vi "Attenuator Unflatten Test Parameters.vi"(9 "error in (no error)":errorcluster, 10 "Parameter String":string) -> (1 "error out":errorcluster, 2 "Attenuator Test Parameters":T2={"Stimulus"={"ATT Stimulus"={"Normalize"=TRUE, "Value (dB)"=0.0}, "VNA Stimulus"={"Use Instrument Settings"=FALSE, "Blank Frequencies"=FALSE, "Sweep Type"=enum."Linear", "Sweep"={"Fstart"=500.0, "Fstop"=1500.0, "Units"=enum."MHz", "Points"=201}, "Power (dBm)"=999.0, "IFBW (Hz)"=-1.0, "Sweep Time (s)"=-1.0, "Calibration"={"State"=FALSE, "String"=""}}}, "Measurement"={"Step (dB)"=enum."0.25", "Start (dB)"=0.0, "Stop (dB)"=31.75}, "Limit"={"Maximum Error"=0.3}, "Normalization"={"Normalized?"=FALSE, "Normalization Values (dB)"=[]}} {"Stimulus"."VNA Stimulus"."Sweep Time (s)" format="%.3g"}, 5 "Test Version":string)   [LabVIEW 2011]
uses:
  TypeDefs/Attenuator Test Parameters.ctl
  TypeDefs/Attenuator Stimulus Parameters.ctl
  TypeDefs/Attenuator ATT Stimulus.ctl
  TypeDefs/Attenuator VNA Stimulus.ctl
  S Parameter/TypeDefs/SP Frequency Units.ctl
  TypeDefs/Attenuator VNA Calibration State.ctl
  TypeDefs/Attenuator Measurement Cluster.ctl
  TypeDefs/Attenuator Limit.ctl
  TypeDefs/Attenuator Calibration State.ctl
  Test Return Parameter.ctl
panel:
  in  "Return Parameter":T1
  out "Parameter Variant":variant
  in  "Required Instruments":string[](array[string])=["ATT", "VNA"]
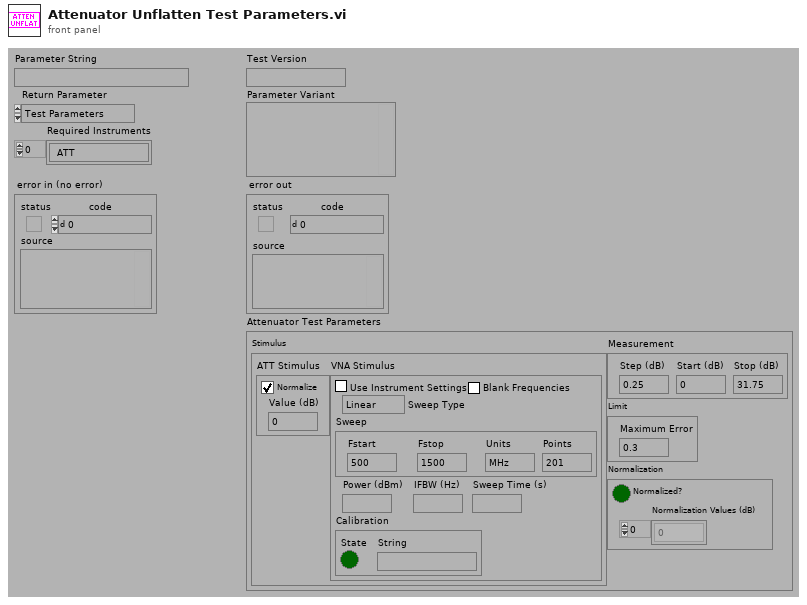
[diagram p1: front panel]
types:
  T1 = typedef "Test Return Parameter.ctl" = enum16{"Test Parameters", "Required Instruments", "Datasheets", "QuickMode"}
  T2 = typedef "Attenuator Test Parameters.ctl" = cluster{"Stimulus":T3, "Measurement":T8, "Limit":T9, "Normalization":T10}
  T3 = typedef "Attenuator Stimulus Parameters.ctl" = cluster{"ATT Stimulus":T4, "VNA Stimulus":T5}
  T4 = typedef "Attenuator ATT Stimulus.ctl" = cluster{"Normalize":bool, "Value (dB)":dbl}
  T5 = typedef "Attenuator VNA Stimulus.ctl" = cluster{"Use Instrument Settings":bool, "Blank Frequencies":bool, "Sweep Type":enum32{"Linear", "Logarithmic", "List", "Power", "CW"}, "Sweep":cluster{"Fstart":dbl, "Fstop":dbl, "Units":T6, "Points":i32}, "Power (dBm)":dbl, "IFBW (Hz)":dbl, "Sweep Time (s)":dbl, "Calibration":T7}
  T6 = typedef "SP Frequency Units.ctl" = enum16{"Hz", "kHz", "MHz", "GHz", "Points"}
  T7 = typedef "Attenuator VNA Calibration State.ctl" = cluster{"State":bool, "String":string}
  T8 = typedef "Attenuator Measurement Cluster.ctl" = cluster{"Step (dB)":enum16{"0.25", "0.50", "1.00"}, "Start (dB)":dbl, "Stop (dB)":dbl}
  T9 = typedef "Attenuator Limit.ctl" = cluster{"Maximum Error":dbl}
  T10 = typedef "Attenuator Calibration State.ctl" = cluster{"Normalized?":bool, "Normalization Values (dB)":dbl[]}
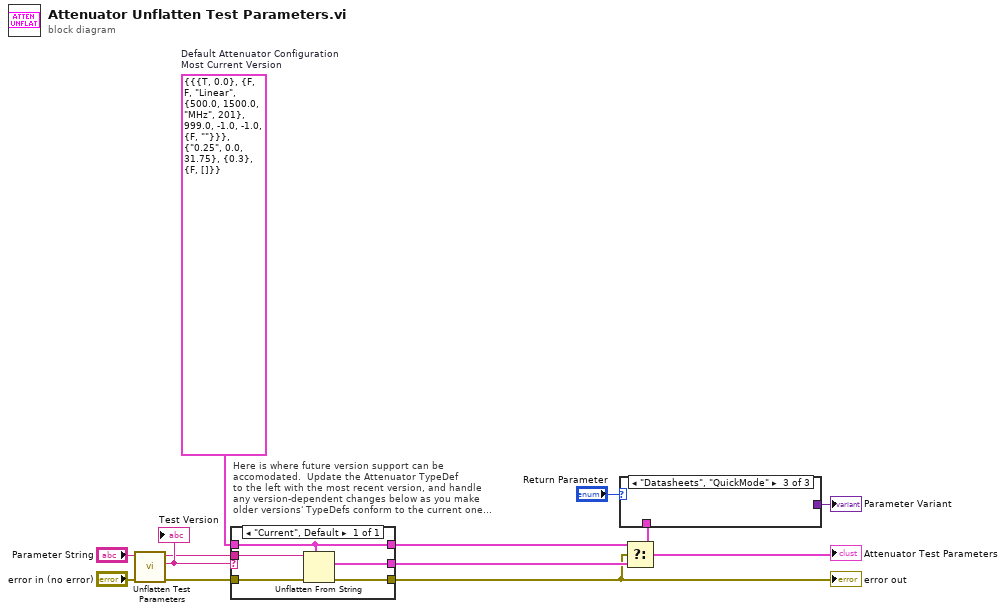
[diagram p0: block diagram]
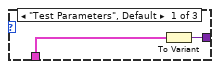
[diagram p2: hidden frame]
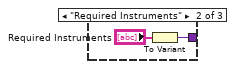
[diagram p3: hidden frame]
diagram:
  w1 = T2 {"Stimulus"={"ATT Stimulus"={"Normalize"=TRUE, "Value (dB)"=0.0}, "VNA Stimulus"={"Use Instrument Settings"=FALSE, "Blank Frequencies"=FALSE, "Sweep Type"=enum."Linear", "Sweep"={"Fstart"=500.0, "Fstop"=1500.0, "Units"=enum."MHz", "Points"=201}, "Power (dBm)"=999.0, "IFBW (Hz)"=-1.0, "Sweep Time (s)"=-1.0, "Calibration"={"State"=FALSE, "String"=""}}}, "Measurement"={"Step (dB)"=enum."0.25", "Start (dB)"=0.0, "Stop (dB)"=31.75}, "Limit"={"Maximum Error"=0.3}, "Normalization"={"Normalized?"=FALSE, "Normalization Values (dB)"=[]}}  # Default Attenuator Configuration Most Current Version
  # "Here is where future version support can be\naccomodated.  Update the Attenuator TypeDef\nto the left with the most recent version, and handle\nany version-dependent changes below as you make\nolder versions' TypeDefs conform to the current one..."
  n1 = call "Unflatten Test Parameters.vi"("error in (no error)"="error in (no error)", "Flattened Test Parameters with Version (\"\")"="Parameter String") -> ("error out"=w3:errorcluster, "Test Version"=w11:string, "Flat Test Parameters"=w10:string)  [unwired: 3 out]
  "Test Version" <- w11
  n2 = case shown="\"Current\", Default" w11 {
    tunnel: [w16] -> w9
    tunnel: w10 -> [w17]
    tunnel: [w14] -> w4
    tunnel: w3 -> [w15]
    tunnel: w1 -> [w13]
    tunnel: [w13] -> w2
    frame "Current", Default {
      n3 = Unflatten From String(type=w13, binary string=w17, error in (no error)=w15) -> (value=w16:T2, error out=w14:errorcluster)  [unwired: 3 out]
    }
  }
  "error out" <- w4
  n4 = Select(t=w2, s=w4, f=w9) -> (s? t:f=w6:T2)
  "Attenuator Test Parameters" <- w6
  n5 = case shown="\"Datasheets\", \"QuickMode\"" "Return Parameter" {
    tunnel: [w19 w21 _] -> w7
    tunnel: w6 -> [w18 _ _]
    frame "Test Parameters", Default {
      n6 = To Variant(anything=w18) -> (Variant=w19:variant)
    }
    frame "Required Instruments" {
      n7 = To Variant(anything="Required Instruments") -> (Variant=w21:variant)
    }
    frame "Datasheets", "QuickMode" {
    }
  }
  "Parameter Variant" <- w7
